vi "AK_Ini_vi.vi"   [LabVIEW 2020, in "Amium PNS.lvlib" / "AK Kommunikation.lvlib"]
uses:
  AK Kommunikation.lvlib
  Amium Kommandos verwalten Aktionen.ctl
types:
  T1 = typedef "Amium PNS.lvlib/AK Kommunikation.lvlib/Amium Kommandos verwalten Aktionen.ctl" = enum16{"lesen", "setzen Ende", "setzen Pos1", "senden", "initalisieren", "prüfen", "Kommandos"}
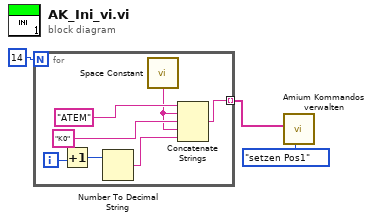
[diagram p0: block diagram]
diagram:
  n1 = for {
    N: 14 -> [_]
    tunnel: [w5] -> w1 mode=indexing
    i -> [w10]
    n2 = Increment(x=w10) -> (x+1=w9:i32)
    n3 = Number To Decimal String(number=w9) -> (decimal integer string=w6:string)  [unwired: 1 in]
    n4 = call <vilib>:"Space Constant.vi"() -> ("String"=w4:string)
    n5 = Concatenate Strings("ATEM", w4, "K0", w4, w6) -> (w5:string)
  }
  n6 = call "Amium Kommandos verwalten.vi"("Aktionen"=Amium_Kommandos_verwalten_Aktionen."setzen Pos1", "neues Kommando Array"=w1) -> ()  [unwired: 7 in, 3 out]
